vi "6510多功能.vi"() -> ()   [LabVIEW 2019]
uses:
  <instrlib>/Keithley DMM6500 DAQ6500 Series/Public/Configure/Configure Temperature (RTD).vi
  <instrlib>/Keithley DMM6500 DAQ6500 Series/Public/Data/Read (Multiple Points).vi
  <instrlib>/Keithley DMM6500 DAQ6500 Series/Keithley DMM6500 DAQ6500 Series.lvlib
panel:
  out "Measurements":dbl[](array[numeric])
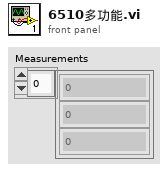
[diagram p1: front panel]
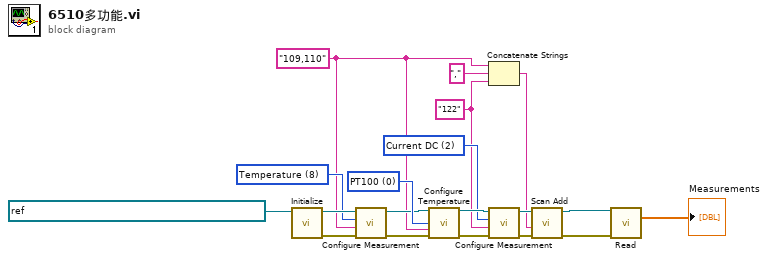
[diagram p0: block diagram]
diagram:
  w2 = "122" ("Channel List(\"\")")
  w5 = 2 items=[" Voltage DC", "Voltage AC", "Current DC", "Current AC", "Resistance", "4-wire Resistance", "Diode", "Capacitance", "Temperature", "Continuity", "Frequency", "Period", "Voltage Ratio"] ("Function (0: Voltage DC)")
  w12 = 8 items=[" Voltage DC", "Voltage AC", "Current DC", "Current AC", "Resistance", "4-wire Resistance", "Diode", "Capacitance", "Temperature", "Continuity", "Frequency", "Period", "Voltage Ratio"] ("Function (0: Voltage DC)")
  w4 = "109,110" ("Channel List(\"\")")
  w18 = 0 items=["PT100", "PT385", "PT3916", "D100", "F100", "USER"] ("RTD Type (0: PT100)")
  n1 = call <instrlib>:"Initialize.vi"("VISA resource name"=refnum<visa-resource-name> "USB0::0x05E6::0x6510::04434284::INSTR") -> ("error out"=w11:errorcluster, "VISA resource name out"=w14:refnum<visa-resource-name>)  [unwired: 9 in]
  n2 = call <instrlib>:"Configure Measurement.vi"("error in (no error)"=w11, "Channel List(\"\")"=w4, "Function (0: Voltage DC)"=w12, "VISA resource name"=w14) -> ("error out"=w10:errorcluster, "VISA resource name out"=w13:refnum<visa-resource-name>)  [unwired: 6 in]
  n3 = call-poly <instrlib>:"Configure Temperature.vi"("VISA resource name"=w13, "RTD Type (0: PT100)"=w18, "Channel List(\"\")"=w4, "error in (no error)"=w10) -> ("VISA resource name out"=w9:refnum<visa-resource-name>, "error out"=w8:errorcluster)  [unwired: 10 in]
  n4 = Concatenate Strings(w4, "," ("字符串"), w2) -> (w1:string)
  n5 = call <instrlib>:"Configure Measurement.vi"("error in (no error)"=w8, "Channel List(\"\")"=w2, "Function (0: Voltage DC)"=w5, "VISA resource name"=w9) -> ("error out"=w7:errorcluster, "VISA resource name out"=w6:refnum<visa-resource-name>)  [unwired: 6 in]
  n6 = call <instrlib>:"Scan Add.vi"("error in (no error)"=w7, "Channel List(\"\")"=w1, "VISA resource name"=w6) -> ("error out"=w16:errorcluster, "VISA resource name out"=w17:refnum<visa-resource-name>)  [unwired: 7 in]
  n7 = call-poly <instrlib>:"Read.vi"("VISA resource name"=w17, "error in (no error)"=w16) -> ("Measurements"=→"Measurements":dbl[])  [unwired: 11 in, 2 out]
